vi "rc_circuit.vi"() -> ()   [LabVIEW 2023]
uses:
  States.ctl
  <vilib>/measure/NI_MAPro.lvlib
  <vilib>/measure/matone.llb/Extract Single Tone Information 1 Chan.vi
  <vilib>/Analysis/NI_AALBase.lvlib
  <vilib>/Analysis/baseanly.llb/Mean (DBL).vi
  <vilib>/Analysis/NI_AALPro.lvlib
  <vilib>/Analysis/6fits.llb/Confidence Interval (Exp).vi
  DAQmxParams.ctl
panel:
  in  "DAQ params":T1 {"Trigger slope" items=["Rising", "Falling"]; "Trigger level" min=-10.0 max=10.0 step=1.0 scale=-10.0..10.0}
  out "DAQ Graph":dbl[](graph)
  in  "Fit Canale":enum16{"Primo", "Secondo", "Terzo"}(ring)
  in  "Analisi Canale":enum16{"Primo", "Secondo", "Terzo"}(ring)
  in  "Pulisci Grafico":bool
  in  "Analisi Frequenza":bool
  out "Analisi in Frequenza":cluster{"X":dbl, "Y":dbl}[](graph)
  in  "Esci":bool
  in  "last points":i32
  in  "Subtract mean of":bool
  out "delta rc":dbl
  out "rc":dbl
  out "Fit esponenziale":cluster{"X":dbl, "Y":dbl}[](graph)
  in  "Canali DAQ":T2(array[cluster]) {"Max value" min=0.0 max=10.0 step=1.0; "Min value" min=-10.0 max=10.0 step=1.0}
  in  "Fit":bool
  in  "DAQ":bool
  # "us"
  # "RC ="
  # "+/-"
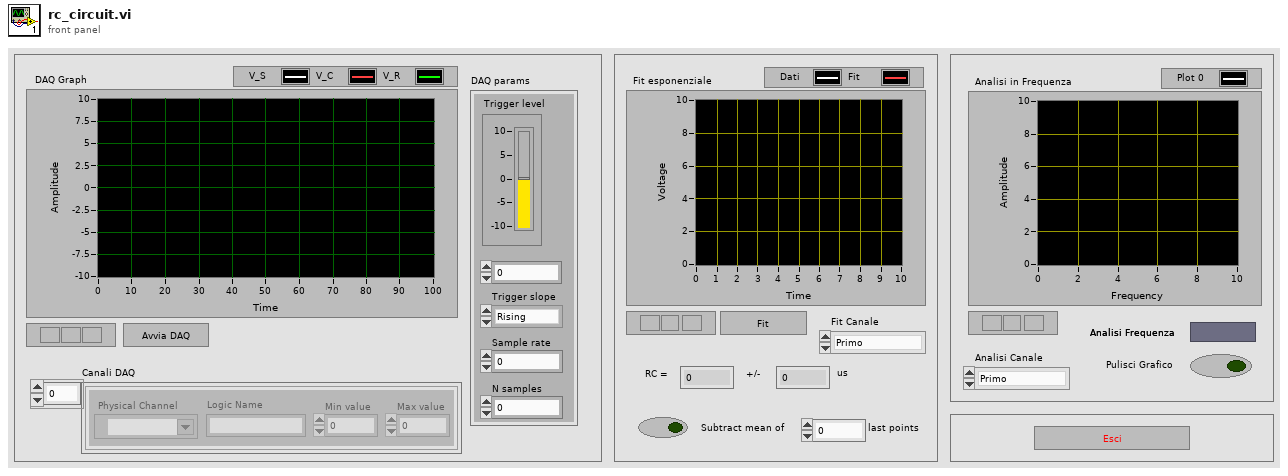
[diagram p1: front panel]
types:
  T1 = typedef "DAQmxParams.ctl" = cluster{"Trigger level":dbl, "Trigger slope":u16, "Sample rate":dbl, "N samples":i32}
  T2 = cluster{" Physical Channel":tag, "Logic Name":string, "Min value":dbl, "Max value":dbl}[]
  T3 = typedef "States.ctl" = enum16{"Idle", "Acquire", "Fit", "Stop"}
  T4 = cluster{"detected frequency":dbl, "detected amplitude":dbl}
  T5 = cluster{"detected frequency":dbl, "detected amplitude":dbl}[]
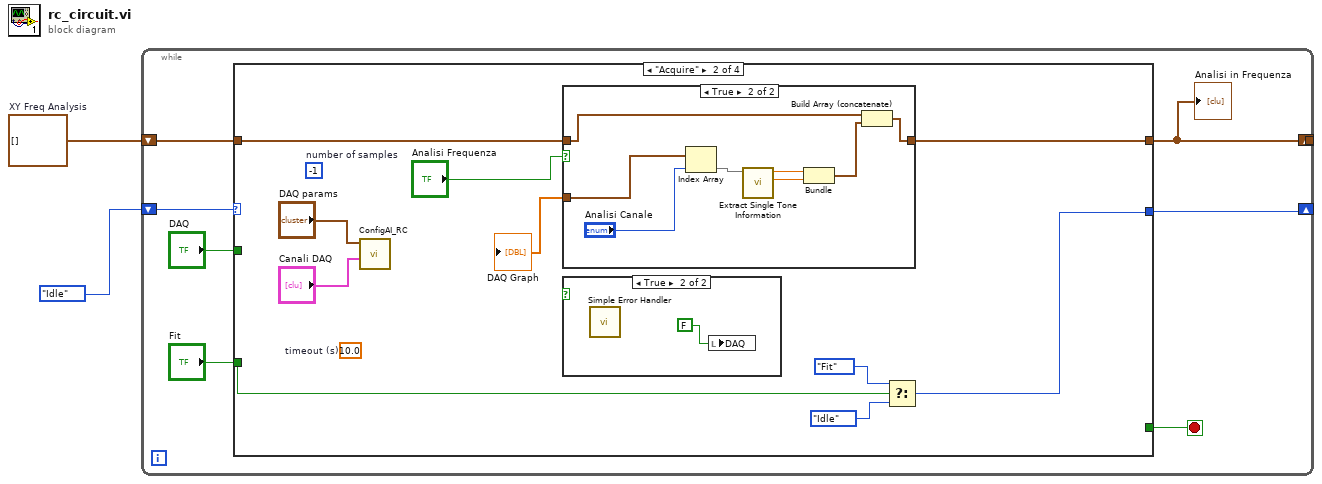
[diagram p0: block diagram]
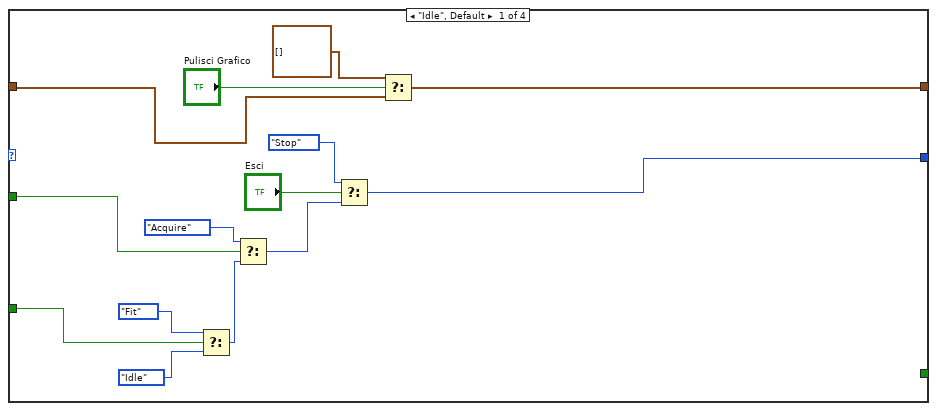
[diagram p2: hidden frame]
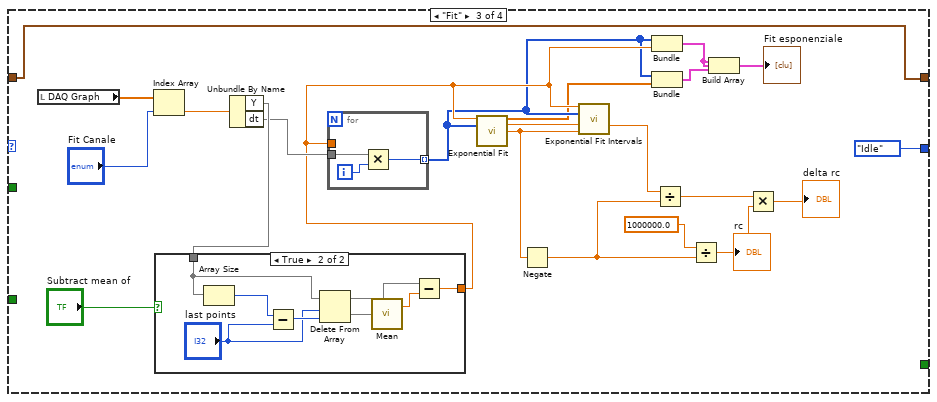
[diagram p5: hidden frame]
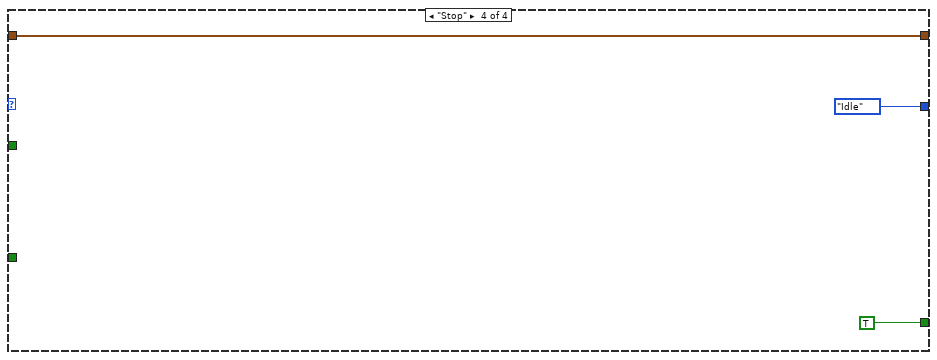
[diagram p7: hidden frame]
diagram:
  w2 = cluster{dbl, dbl}[] []  # XY Freq Analysis
  n1 = while {
    shift-right: [w5] -> _
    shift-left: States."Idle" ("Enum") -> [w7]
    tunnel: [w4] -> _
    shift-right: _ -> [_]
    shift-left: w2 -> [w6]
    stop <- w3 stop-if-true
    n2 = case shown="\"Acquire\"" w7 {
      tunnel: "DAQ" -> [w13 _ _ _]
      tunnel: "Fit" -> [w14 w33 _ _]
      tunnel: w6 -> [w11 w31 w45 w75]
      tunnel: [w17 w32 States."Idle" ("Enum") States."Idle" ("Enum")] -> w5
      tunnel: [w10 w30 w45 w75] -> w4
      tunnel: [_ _ _ TRUE] -> w3
      frame "Idle", Default {
        n3 = Select(t=States."Fit" ("Enum"), s=w14, f=States."Idle" ("Enum")) -> (s? t:f=w20:T3)
        n4 = Select(t=States."Acquire" ("Enum"), s=w13, f=w20) -> (s? t:f=w23:T3)
        n5 = Select(t=States."Stop" ("Enum"), s="Esci", f=w23) -> (s? t:f=w17:T3)
        n6 = Select(t=cluster{dbl, dbl}[] [] ("XY Freq Analysis"), s="Pulisci Grafico", f=w11) -> (s? t:f=w10:cluster{dbl, dbl}[])
      }
      frame "Acquire" {
        (unwired) -1  # number of samples
        (unwired) 10.0  # timeout (s)
        n7 = call "ConfigAI_RC.vi"("DAQmx Channel Specs"="Canali DAQ", "DAQ params"="DAQ params") -> ()  [unwired: 9 in, 1 out]
        n8 = case shown="True" "Analisi Frequenza" {
          tunnel: w31 -> [_ w42]
          tunnel: [_ w41] -> w30
          tunnel: "DAQ Graph" -> [_ w35]
          frame False {
          }
          frame True {
            n9 = Index Array(array=w35, index="Analisi Canale") -> (element=w37)
            n10 = call-poly <vilib>:"Extract Single Tone Information.vi"("time signal in"=w37) -> ("detected amplitude"=w38:dbl, "detected frequency"=w39:dbl)  [unwired: 5 in, 4 out]
            n11 = Bundle("detected frequency"=w39, "detected amplitude"=w38) -> (w40:T4)  [unwired: 1 in]
            n12 = Build Array (concatenate)(w42, w40) -> (w41:T5)
          }
        }
        n13 = case shown="True" {
          selector: _ -> [_ _]
          frame False {
          }
          frame True {
            n14 = call <vilib>:"Simple Error Handler.vi"() -> ()  [unwired: 5 in, 5 out]
            n15 = local write "DAQ"(FALSE) -> ()
          }
        }
        n16 = Select(t=States."Fit" ("Enum"), s=w33, f=States."Idle" ("Enum")) -> (s? t:f=w32:T3)
      }
      frame "Fit" {
        n17 = local read "DAQ Graph"() -> (w43:dbl[])
        n18 = Index Array(array=w43, index="Fit Canale") -> (element=w62:dbl)
        n19 = Unbundle By Name(w62) -> ("Y"=w60, "dt"=w59)
        n20 = case shown="True" "Subtract mean of" {
          tunnel: w60 -> [_ w70]
          tunnel: [_ w74] -> w51
          frame False {
          }
          frame True {
            n21 = Array Size(array=w70) -> (size(s)=w68:i32)
            n22 = Subtract(x=w68, y="last points") -> (x-y=w69:i32)
            n23 = Delete From Array(array=w70, length="last points", index=w69) -> (deleted portion=w72, array with subset deleted=w73)
            n24 = call-poly <vilib>:"Mean.vi"("X"=w72) -> ("mean"=w71:dbl)  [unwired: 1 out]
            n25 = Subtract(x=w73, y=w71) -> (x-y=w74:dbl)
          }
        }
        n26 = for {
          tunnel: w59 -> [w65]
          tunnel: w51 -> [_]
          tunnel: [w64] -> w50 mode=indexing
          i -> [w66]
          n27 = Multiply(x=w65, y=w66) -> (x*y=w64:i32)
        }
        n28 = call <vilib>:"Exponential Fit.vi"("Y"=w51, "X"=w50) -> ("Best Exponential Fit"=w49:dbl[], "amplitude"=w58:dbl, "damping"=w44:dbl)  [unwired: 8 in, 3 out]
        n29 = Negate(x=w44) -> (-x=w56:dbl)
        n30 = call-poly <vilib>:"Exponential Fit Intervals.vi"("Y"=w51, "X"=w50, "amplitude"=w58, "damping"=w44) -> ("delta damping"=w53:dbl)  [unwired: 7 in, 4 out]
        n31 = Bundle(w50, w51) -> (w47:cluster{i32[], dbl})  [unwired: 1 in]
        "Fit esponenziale" <- w47
        n32 = Bundle(w50, "Best Exponential Fit"=w49) -> (w48:cluster{i32[], "Best Exponential Fit":dbl[]})  [unwired: 1 in]
        n33 = Divide(x=w53, y=w56) -> (x/y=w54:dbl)
        n34 = Divide(x=1000000.0, y=w56) -> (x/y=w55:dbl)
        "rc" <- w55
        n35 = Build Array(w47, w47, w48) -> ()
        n36 = Multiply(x=w54, y=w55) -> (x*y=→"delta rc":dbl)
      }
      frame "Stop" {
      }
    }
    "Analisi in Frequenza" <- w4
  }
